vi "Delay Timer.vi"(0 "delay time(ms)":u32=3724, 1 "ref stop btn":refnum<vi>) -> ()   [LabVIEW 2018]
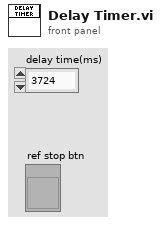
[diagram p1: front panel]
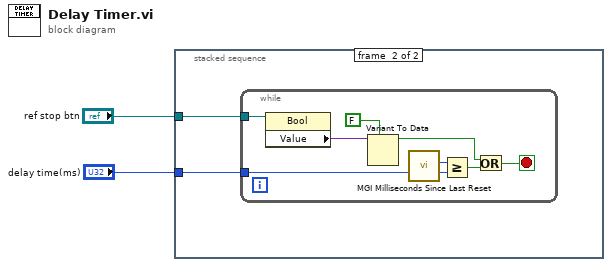
[diagram p0: block diagram]
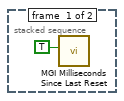
[diagram p2: hidden frame]
diagram:
  n1 = stacked-sequence {
    tunnel: "ref stop btn" -> [_ w5]
    tunnel: "delay time(ms)" -> [_ w4]
    frame #0 {
      n2 = call <userlib>:"MGI Milliseconds Since Last Reset.vi"("Reset (F)"=TRUE) -> ()  [unwired: 5 in, 2 out]
    }
    frame #1 {
      n3 = while {
        tunnel: w4 -> [w13]
        tunnel: w5 -> [w11]
        stop <- w7 stop-if-true
        n4 = property class="Bool"(reference=w11) -> ("Value"=w10:variant)  [unwired: 1 in, 2 out]
        n5 = Variant To Data(type=FALSE, Variant=w10) -> (data=w6:bool)  [unwired: 1 in, 1 out]
        n6 = call <userlib>:"MGI Milliseconds Since Last Reset.vi"() -> ("ms"=w12:u32)  [unwired: 6 in, 1 out]
        n7 = Greater Or Equal?(x=w12, y=w13) -> (x >= y?=w8:bool)
        n8 = Or(x=w6, y=w8) -> (x .or. y?=w7:bool)
      }
    }
  }
